vi "ReadControllerInformation.vi"(0 "System no.":i32, 5 "error in (no error)":errorcluster) -> (10 "Identification":string, 11 "HLP? answer":string, 14 "Connected Axes":string[](array[string]), 16 "Stage names":string[](array[string]), 19 "error out":errorcluster)   [LabVIEW 2020]
uses:
  ProgramData/PI/LabVIEW/Low Level/Support.llb/HasCommand?.vi
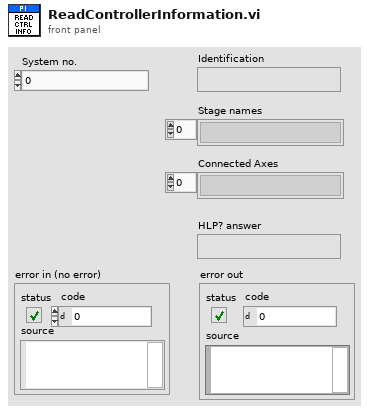
[diagram p1: front panel]
types:
  T1 = typedef "Controller names.ctl" = enum16{"None", "Analog", "C-702", "C-413", "C-414", "C-843", "C-843.PM", "C-844", "C-848", "C-865", "C-866", "C-867", "C-877", "C-880", "C-884", "C-885", "C-886", "C-887", "C-891", "E-135", "E-516", "E-517", "E-518", "E-709", "E-710", "E-712", "E-725", "E-727", "E-753", "E-754", "E-755", "E-761", "E-816", "E-861", "E-870", "E-871", "E-872", "E-873", "E-874", "F-206", "HydraPollux", "M-840", "M-850", "M-8X0", "Mercury", "Mercury_GCS", "PI_GCS2"}
  T2 = typedef "Syntax.ctl" = enum16{"GCS 1.0", "GCS 2.0", "GCS 3.0"}
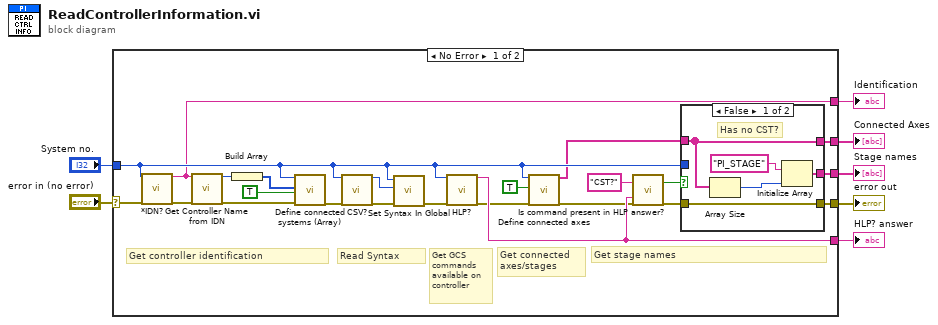
[diagram p0: block diagram]
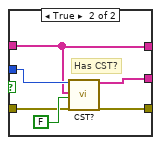
[diagram p2: hidden frame]
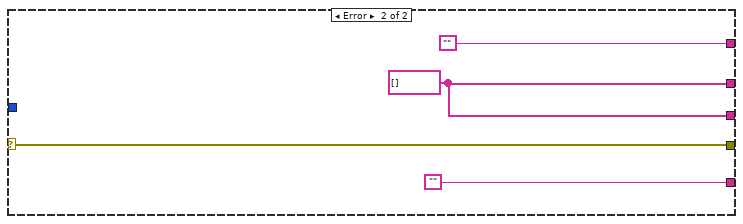
[diagram p3: hidden frame]
diagram:
  n1 = case shown="No Error" "error in (no error)" {
    selector: "error in (no error)" -> [w11 w45]
    tunnel: "System no." -> [w28 _]
    tunnel: [w25 "" ("Help string")] -> w6
    tunnel: [w9 w44] -> w5
    tunnel: [w19 w45] -> w4
    tunnel: [w13 w44] -> w3
    tunnel: [w8 ""] -> w1
    frame No Error {
      # "Read Syntax"
      # "Get stage names"
      # "Get connected \naxes/stages"
      # "Get GCS commands \navailable on controller"
      # "Get controller identification"
      n2 = call "*IDN?.vi"("System no."=w28, "error in"=w11) -> ("Identification"=w8:string, "error out"=w16:errorcluster)  [unwired: 16 out]
      n3 = call "Get Controller Name from IDN.vi"("Identification"=w8, "error in"=w16) -> ("Controller Name"=w18:T1, "error out"=w17:errorcluster)  [unwired: 16 out]
      n4 = Build Array(w18) -> (w15:T1[])
      n5 = call "Define connected systems (Array).vi"("System no."=w28, "Controller names"=w15, "Change only one system?"=TRUE, "error in"=w17) -> ("error out"=w26:errorcluster)  [unwired: 15 out]
      n6 = call "CSV?.vi"("System no."=w28, "error in"=w26) -> ("Syntax"=w27:T2, "error out"=w29:errorcluster)  [unwired: 16 out]
      n7 = call "Set Syntax In Global.vi"("error in"=w29, "Syntax"=w27, "System no."=w28) -> ("error out"=w30:errorcluster)  [unwired: 8 in]
      n8 = call "HLP?.vi"("System no."=w28, "error in"=w30) -> ("Help string"=w25:string, "error out"=w20:errorcluster)  [unwired: 16 out]
      n9 = call "Define connected axes.vi"("System no."=w28, "Read from\ncontroller?"=TRUE ("Read from\ncontroller?"), "error in"=w20) -> ("Conn. Axes out"=w10:string[], "error out"=w23:errorcluster)  [unwired: 2 in, 13 out]
      n10 = call-poly "Is command present in HLP answer?.vi"("Command"="CST?" ("String"), "HLP? answer"=w25, "error in"=w23) -> ("Is command available?"=w21:bool, "error out"=w24:errorcluster)  [unwired: 2 in, 13 out]
      n11 = case shown="False" w21 {
        tunnel: [w33 w41] -> w13
        tunnel: [w35 w39] -> w19
        tunnel: w24 -> [w35 w38]
        tunnel: w28 -> [_ w37]
        tunnel: w10 -> [w31 w36]
        tunnel: [w31 w36] -> w9
        frame False {
          # "Has no CST?"
          n12 = Array Size(array=w31) -> (size(s)=w32:i32)
          n13 = Initialize Array("PI_STAGE", w32) -> (w33:string[])
        }
        frame True {
          # "Has CST?"
          n14 = call "CST?.vi"("System no."=w37, "Axes to query"=w36, "All Axes?"=FALSE, "error in"=w38) -> ("Stage names"=w41:string[], "error out"=w39:errorcluster)  [unwired: 1 in, 13 out]
        }
      }
    }
    frame Error {
      w44 = string[] [] ("Stage names")
    }
  }
  "HLP? answer" <- w6
  "Connected Axes" <- w5
  "error out" <- w4
  "Stage names" <- w3
  "Identification" <- w1
